vi "Check Device Name.vi"(8 "error in (no error)":errorcluster, 9 "New Name":string, 10 "Device":refnum<class "Device.lvclass">, 11 "HAL Editor in":refnum<class "HAL Editor.lvclass">) -> (0 "error out":errorcluster, 2 "Valid?":bool, 3 "HAL Editor out":refnum<class "HAL Editor.lvclass">)   [LabVIEW 2020, in "HAL Config.lvlib" / "HAL Editor.lvclass"]
uses:
  HAL Editor.lvclass
  build/ppl/lv-hal.lvlibp/Device/Device.lvclass
  HAL Editor.lvclass/HAL Editor.ctl
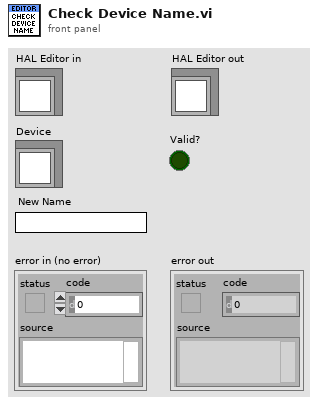
[diagram p1: front panel]
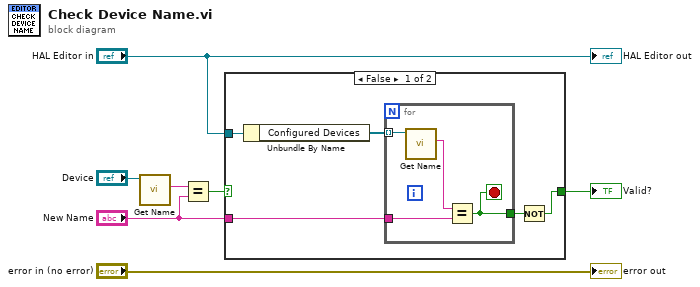
[diagram p0: block diagram]
diagram:
  n1 = call "Get Name.vi"("Device in"="Device") -> ("Name"=w5:string)  [unwired: 8 in, 2 out]
  n2 = Equal?(x=w5, y="New Name") -> (x = y?=w4:bool)
  n3 = case shown="False" w4 {
    selector: w4 -> [_ w17]
    tunnel: [w8 w17] -> w3
    tunnel: "New Name" -> [w10 _]
    tunnel: "HAL Editor in" -> [w12 _]
    frame False {
      n4 = Unbundle By Name(w12) -> ("Configured Devices"=w11:refnum<class "Device.lvclass">[])
      n5 = for {
        tunnel: w11 -> [w16] mode=indexing
        tunnel: w10 -> [w15]
        tunnel: [w13] -> w9
        stop <- w13 stop-if-true
        n6 = call "Get Name.vi"("Device in"=w16) -> ("Name"=w14:string)  [unwired: 8 in, 2 out]
        n7 = Equal?(x=w14, y=w15) -> (x = y?=w13:bool)
      }
      n8 = Not(x=w9) -> (.not. x?=w8:bool)
    }
    frame True {
    }
  }
  "Valid?" <- w3
  "error out" <- "error in (no error)"
  "HAL Editor out" <- "HAL Editor in"
